vi "XML getApiResponse.vi"(11 "Formatted XML":string) -> (3 "PIM API Response":T1={"#attributes"={"xmlns"="http://www.summitekinstruments.com", "xmlns:xsi"="http://www.w3.org/2001/XMLSchema-instance", "xsi:schemaLocation"="http://www.summitekinstruments.com PIMXMLSchema.xsd"}, "Responses"={"#attributes"={"Legacy"=FALSE}, "Response"=[]}})   [LabVIEW 2011]
uses:
  Controls/PIM.API.RESPONSE.ctl
  Controls/PIM.API.Response.Collection.ctl
  Controls/PIM.API.Response.Unique.ctl
  Controls/PIM.API.Response.Samples.ctl
  iQA Sweep Behavior.ctl
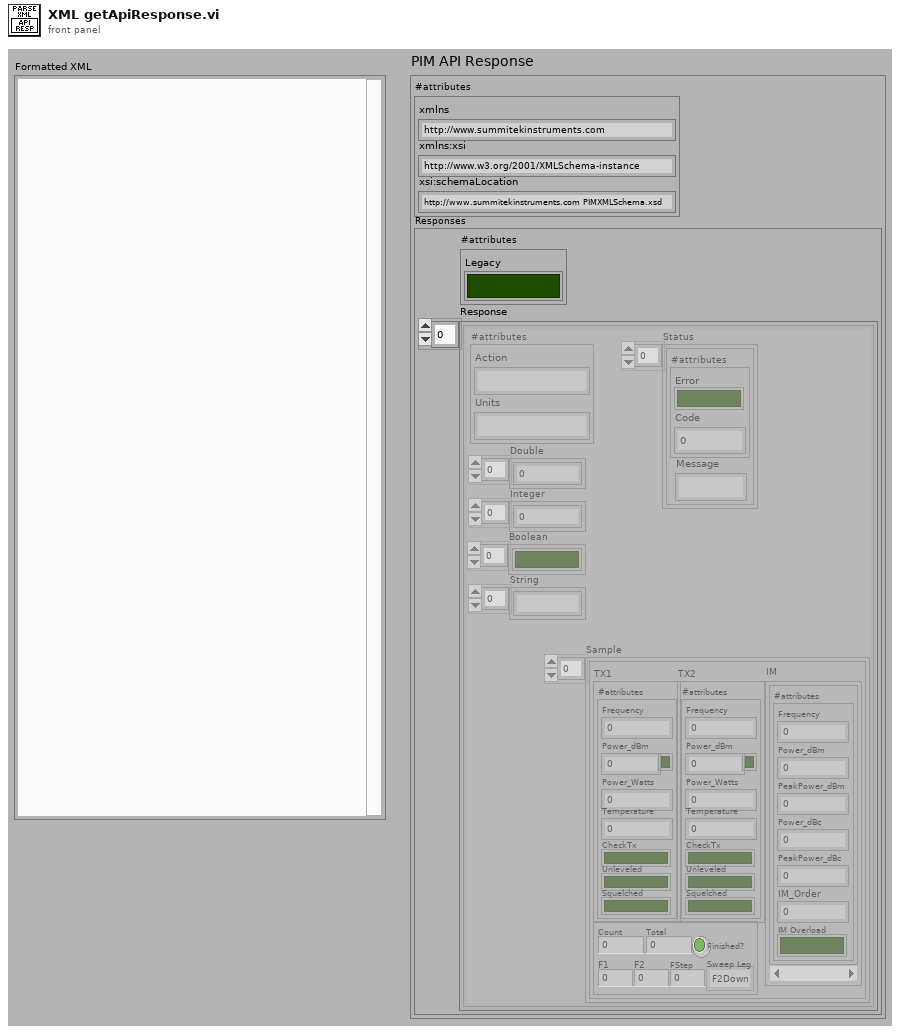
[diagram p1: front panel]
types:
  T1 = typedef "PIM.API.RESPONSE.ctl" = cluster{"#attributes":cluster{"xmlns":string, "xmlns:xsi":string, "xsi:schemaLocation":string}, "Responses":T2}
  T2 = typedef "PIM.API.Response.Collection.ctl" = cluster{"#attributes":cluster{"Legacy":bool}, "Response":T3[]}
  T3 = typedef "PIM.API.Response.Unique.ctl" = cluster{"#attributes":cluster{"Action":string, "Units":string}, "Double":dbl[], "Integer":i32[], "Boolean":bool[], "String":string[], "Sample":T4[], "Status":cluster{"#attributes":cluster{"Error":bool, "Code":i32}, "Message":string}[]}
  T4 = typedef "PIM.API.Response.Samples.ctl" = cluster{"TX1":cluster{"#attributes":cluster{"Frequency":dbl, "Power_dBm":dbl, "Power_Watts":dbl, "CheckTx":bool, "Unleveled":bool, "Squelched":bool, "Temperature":dbl, "ToneOn":bool}}, "TX2":cluster{"#attributes":cluster{"Frequency":dbl, "Power_dBm":dbl, "Power_Watts":dbl, "CheckTx":bool, "Unleveled":bool, "Squelched":bool, "Temperature":dbl, "ToneOn":bool}}, "IM":cluster{"#attributes":cluster{"Frequency":dbl, "Power_dBm":dbl, "PeakPower_dBm":dbl, "Power_dBc":dbl, "PeakPower_dBc":dbl, "IM_Order":u8, "IM Overload":bool}}[], "#attributes":cluster{"Count":u32, "Total":u32, "Finished?":bool, "Sweep Leg":T5, "F1":dbl, "F2":dbl, "FStep":dbl}}
  T5 = typedef "iQA Sweep Behavior.ctl" = enum16{"F2Down", "F1Up", "RxMultiIM"}
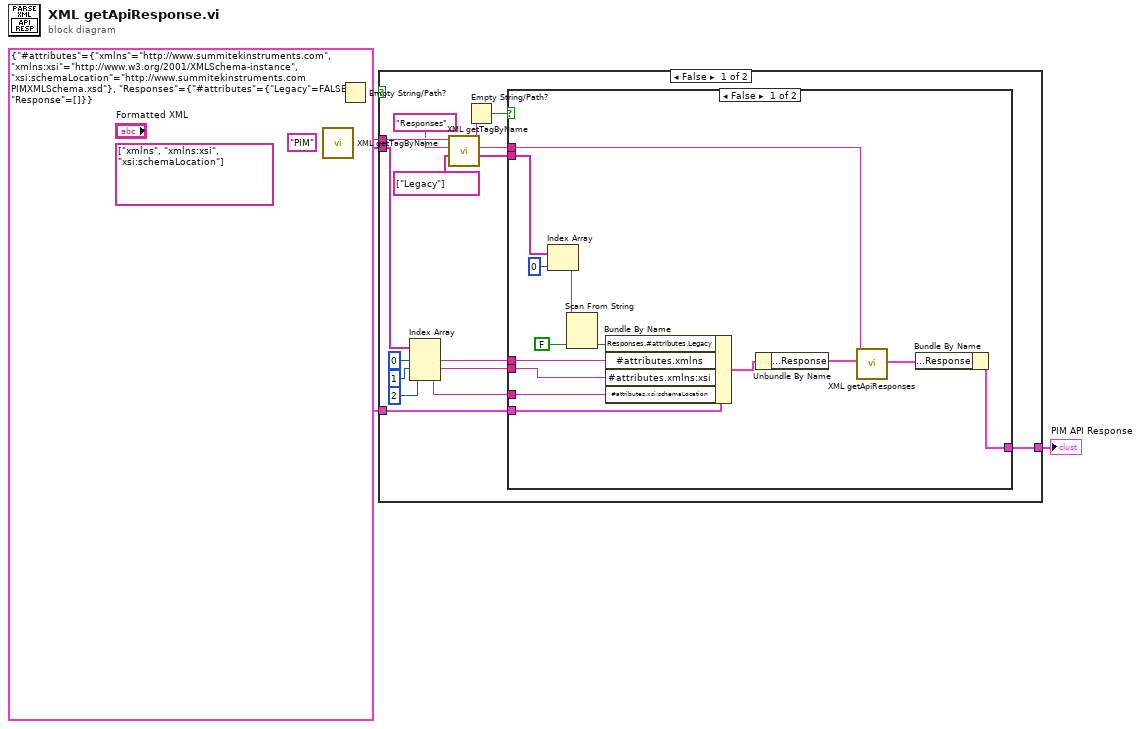
[diagram p0: block diagram]
diagram:
  n1 = call "XML getTagByName.vi"("Get Attributes"=string[] ["xmlns", "xmlns:xsi", "xsi:schemaLocation"], "Tag Name"="PIM", "XML String"="Formatted XML") -> ("Attribute Values"=w3:string[], "Tag Contents"=w2:string, "Matching Tag"=w1:string)  [unwired: 4 in, 2 out]
  n2 = Empty String/Path?(string/path=w1) -> (empty?=w9:bool)
  n3 = case shown="False" w9 {
    tunnel: T1 {"#attributes"={"xmlns"="http://www.summitekinstruments.com", "xmlns:xsi"="http://www.w3.org/2001/XMLSchema-instance", "xsi:schemaLocation"="http://www.summitekinstruments.com PIMXMLSchema.xsd"}, "Responses"={"#attributes"={"Legacy"=FALSE}, "Response"=[]}} ("PIM") -> [w17 w41]
    tunnel: [w10 w41] -> w7
    tunnel: w2 -> [w25 _]
    tunnel: w3 -> [w21 _]
    frame False {
      n4 = Index Array(array=w21, index #1=0 ("index"), index #2=1 ("index"), index #3=2 ("index")) -> (element #1=w20:string, element #2=w19:string, element #3=w18:string)
      n5 = call "XML getTagByName.vi"("Get Attributes"=string[] ["Legacy"], "Tag Name"="Responses", "XML String"=w25) -> ("Attribute Values"=w13:string[], "Tag Contents"=w23:string, "Matching Tag"=w12:string)  [unwired: 4 in, 2 out]
      n6 = Empty String/Path?(string/path=w12) -> (empty?=w11:bool)
      n7 = case shown="False" w11 {
        tunnel: w23 -> [w26 _]
        tunnel: w20 -> [w39 _]
        tunnel: w19 -> [w38 _]
        tunnel: w18 -> [w37 _]
        tunnel: w17 -> [w36 w40]
        tunnel: w13 -> [w30 _]
        tunnel: [w27 w40] -> w10
        frame False {
          n8 = Index Array(array=w30, index=0) -> (element=w33:string)
          n9 = Scan From String(input string=w33, default 1=FALSE ("Legacy")) -> (output 1=w32:bool)  [unwired: 3 in, 3 out]
          n10 = Bundle By Name(cluster=w36, "Responses.#attributes.Legacy"=w32, "#attributes.xmlns"=w39, "#attributes.xmlns:xsi"=w38, "#attributes.xsi:schemaLocation"=w37) -> (w29:T1)
          n11 = Unbundle By Name(w29) -> ("Responses.Response"=w31:T3[])
          n12 = call "XML getApiResponses.vi"("Responses In"=w31, "Responses XML"=w26) -> ("Responses Out"=w28:T3[])  [unwired: 9 in]
          n13 = Bundle By Name(cluster=w29, "Responses.Response"=w28) -> (w27:T1)
        }
        frame True {
        }
      }
    }
    frame True {
      # "Tag Not Found"
    }
  }
  "PIM API Response" <- w7
